vi "Selection ActionBuilder sections.vi"(6 "EC Query Array":T1[](array[typedef])=[enum."Is the EC Backing Pump ON?", enum."Does the EC Backing Pump have a fault?"], 7 "LB Query Array":T1[](array[typedef])=[enum."Is the LB Backing Pump ON?", enum."Does the LB Backing Pump have a fault?"], 9 "EC Command Array":T2[](array[typedef]), 10 "Chamber Selection":T3, 11 "LB Command Array":T2[](array[typedef])) -> (0 "Query Array out":T1[](array[typedef]), 3 "Command Array out":T2[](array[typedef]))   [LabVIEW 2011]
uses:
  Chamber Selection_typdef.ctl
  command_typdef.ctl
  action_typdef.ctl
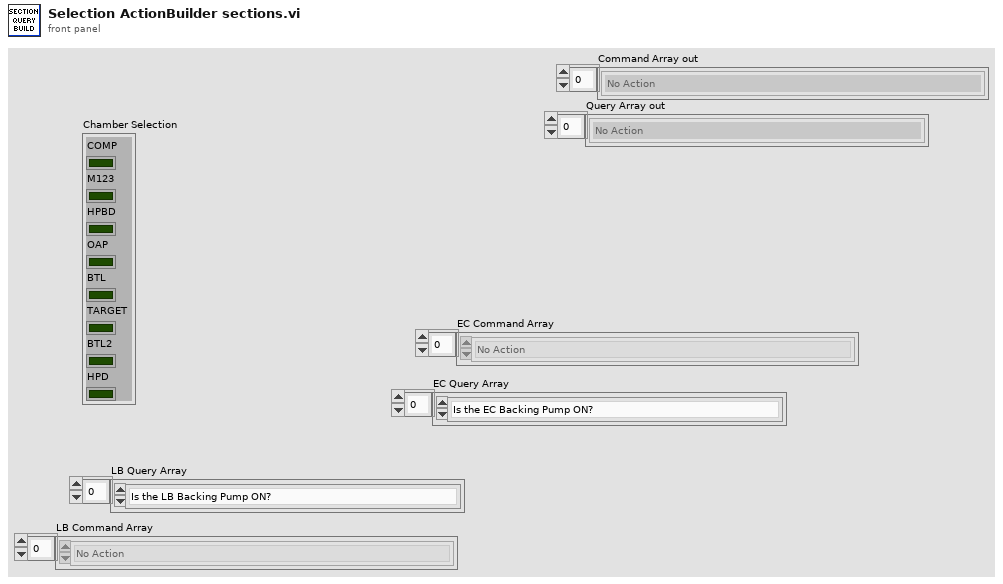
[diagram p1: front panel]
types:
  T1 = typedef "action_typdef.ctl" = enum16{"No Action", "Is EC GPM Mode ON?", "Is EC GPM Mode Off?", "Is EC GVM Mode ON?", "Is EC GVM Off?", "Is  EC GPM or GVM Mode ON?", "Is LB GPM Mode ON?", "Is LB GPM Mode Off?", "Is LB GVM Mode ON?", "Is LB GVM Mode Off?", "Is  LB GPM or GVM Mode ON?", "Is M123 Turbo Gate Valve Opened? ", "Is M123 Turbo Gate Valve Closed?", "Is OAP Turbo Gate Valve Opened?", "Is OAP Turbo Gate Valve Closed?", "Is BTLTurbo Gate Valve Opened?", "Is BTL Turbo Gate Valve Closed?", "Is TARGET Turbo Gate Valve 1Opened?", "Is TARGET1 Turbo Gate Valve Closed?", "Is TARGET Turbo Gate Valve 2 Opened?", "Is TAREGT2 Turbo Gate Valve Closed?", "Is BTL2 Turbo Gate Valve Opened?", "Is BTL2 Turbo Gate Valve Closed?", "Is HPD Turbo Gate Valve Opened?", "Is HPD Turbo Gate Valve Closed?", "Is COMP to M123 gate Valve Opened?", "Is COMP to M123 Valve Closed?", "Is HPBD Gate Valve Opened?", "Is HPBD Gate Valve Closed?", "Is M123 to OAP gate valve opened?", "Is M123 to OAP gate valve closed?", "Is OAP to BLT gate valve opened?", "Is OAP to BTL Gate Valve Closed?", "Is BLT to TARGET gate valve opened?", "Is BTL to TARGET Gate Valve Closed?", "Is TARGET to BLT2 gate valve opened?", "Is TARGET to BTL2 Gate Valve Closed?", "Is BLT2 to HPD gate valve opened?", "Is BTL2 to HPD Gate Valve Closed?", "Is COMP at Atmospheric Pressure?", "Is M123 at Atmospheric Pressure?", "Is BeamDump at Atmospheric Pressure?", "Is OAP at Atmospheric Pressure?", "Is BLT at Atmospheric Pressure", "Is TARGET at Atmospheric Pressure?", "Is BLT2 at Atmospheric Pressure?", "Is HPD at Atmospheric Pressure?", "Is the EC Roughing Pump ON?", "Is the EC Roughing Pump OFF?", "Does the EC Roughing Pump have a fault?", "Is the LB Roughing Pump ON?", "Is the LB Roughing Pump Off?", "Does the LB Roughing Pump have a fault?", "Is the EC Backing Pump ON?", "Is the EC Backing Pump OFF?", "Is the LB Backing Pump ON?", "Is the LB Backing Pump OFF?", "Does the EC Backing Pump have a fault?", "Does the LB Backing Pump have a fault?", "Is the EC Backing Pipe at Atmospheric Pressure", "Is the LB Backing Pipe at Atmospheric Pressure", "Is the EC Backing Manifold at Atmospheric Pressure", "s the LB Backing Manifold at Atmospheric Pressure?", "Is the EC Roughing Pipe at Atmospheric Pressure", "Is the LB Roughing Pipe at Atmospheric Pressure?", "Is the EC Roughing Manifold at Atmospheric Pressure", "Is the LB Roughing Manifold at Atmospheric Pressure", "Is LB Backing Manifold Valve Opened?", "Is EC Backing Manifold Valve Opened?", "Is LB Roughing Manifold Valve Opened?", "Is EC Roughing Manifold Valve Opened?", "Is COMP Roughing Valve Opened?", "Is M123 Roughing Valve Opened?", "Is M123 Roughing Valve Closed?", "Is OAP Roughing Valve Opened?", "Is OAP Roughing Valve Closed?", "Is HPBD Roughing Valve Opened?", "Is HPBD Roughing Valve Closed?", "Is BTL Roughing Valve Opened?", "Is BTL Roughing Valve Closed?", "Is TARGET Roughing Valve Opened?", "Is TARGET Roughing Valve Closed?", "Is BTL2 Roughing Valve Opened?", "Is BTL2 Roughing Valve Closed?", "Is HPD Roughing Valve Opened?", "Is HPD Roughing Valve Closed?", "Is COMP Turbo Backing Valve Opened?", "Is M123 Turbo Backing Valve Opened", "Is HPBD Turbo Backing Valve Opened?", "Is OAP Turbo Backing Valve Opened?", "Is BTL Turbo Backing Valve Opened?", "Is TARGET1 Turbo Backing Valve Opened?", "Is TARGET2 Turbo Backing Valve Opened?", "Is BTL2 Turbo Backing Valve Opened?", "Is HPD Turbo Backing Valve Opened?", "Is M123 Backing at MID-VAC?", "Is OAP Backing at MID-VAC?", "Is TARGET1 Backing at MID-VAC?", "Is TARGET2 Backing at MID-VAC?", "Is BTL Backing at MID-VAC?", "Is BTL2 Backing at MID-VAC?", "Is HPD Backing at MID-VAC?", "Is M123 Turbo in Normal Operation", "Is COMP Turbo in Normal Operation", "Is OAP Turbo in Normal Operation", "Is BTL Turbo in Normal Operation", "Is TARGET1 Turbo in Normal Operation", "Is TARGET2 Turbo in Normal Operation", "Is BTL2 Turbo in Normal Operation", "Is HPD Turbo in Normal Operation", "Is M123 at MID-VAC?", "Is OAP at MID-VAC?", "Is COMP at MID-VAC?", "Is BTL at MID-VAC?", "Is TARGET at MID-VAC?", "Is BTL2 at MID-VAC?", "Is HPD at MID-VAC?"}
  T2 = typedef "command_typdef.ctl" = enum16{"No Action", "Set GPM Mode LB", "EXIT GPM Mode LB", "Set GPM Mode EC", "EXIT GPM Mode EC", "Set GVM mode LB", "Set GVM Mode EC", "Open LB Backing Valve", "Open EC Backing Valve", "Open EC Roughing Valve", "Open LB Roughing Valve", "Open M123 Roughing Valve", "Close M123 Roughing Valve", "Open Compressor Roughing Valve", "Close Compressor Roughing Valve", "Open BeamDump Roughing Valve", "Close BeamDump Roughing Valve", "Open OAP Roughing Valve", "Close OAP Roughing Valve", "Open BTL Roughing Valve", "Close BTL Roughing Valve", "Open Target Roughing Valve", "Close Target Roughing Valve", "Open BTL2 Roughing Valve", "Close BTL2 Roughing Valve", "Open HPD Roughing Valve", "Close HPD Roughing Valve", "LB Start Roughing Pump ", "EC Start Roughing Pump", "Open COMP Turbo Backing Valve", "Open M123 Turbo Backing Valve", "Open OAP Turbo Backing Valve", "Open HPBD Turbo Backing Valve", "Open BLT Turbo Backing Valve", "Open TARGET1 Turbo Backing Valve", "Open TARGET2 Turbo Backing Valve", "Open BLT2 Turbo Backing Valve", "Open HPD Turbo Backing Valve", "LB Start Turbo Backing Pump", "EC Start Turbo Backing Pump", "Start COMP Turbo Pump", "Start M123 Turbo Pump", "Start OAP Turbo Pump", "Start BTL Turbo Pump", "Start TARGET1 Turbo Pump", "Start TARGET2 Turbo Pump", "Start BTL2 Turbo Pump", "Start HPD Turbo Pump", "Open COMP Turbo Gate Valve", "Open M123 Turbo Gate Valve", "Open OAP Turbo Gate Valve", "Open BTL Turbo Gate Valve", "Open TARGET1 Turbo Gate Valve", "Open TARGET2 Turbo Gate Valve", "Open BTL2 Turbo Gate Valve", "Open HPD Turbo Gate Valve"}
  T3 = typedef "Chamber Selection_typdef.ctl" = cluster{"COMP":bool, "M123":bool, "HPBD":bool, "OAP":bool, "BTL":bool, "TARGET":bool, "BTL2":bool, "HPD":bool}
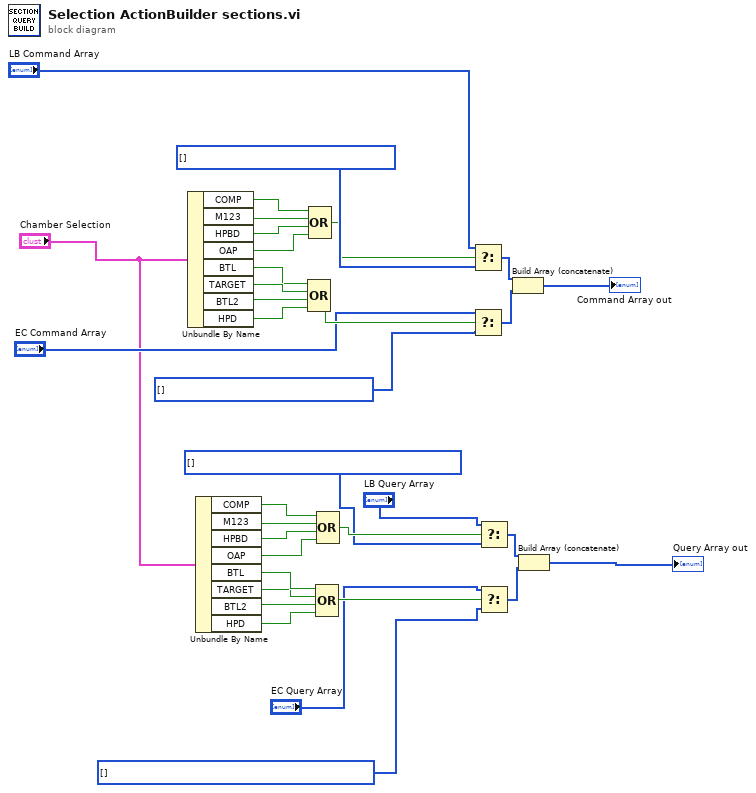
[diagram p0: block diagram]
diagram:
  w2 = T1[] [] items=["No Action", "Is EC GPM Mode ON?", "Is EC GPM Mode Off?", "Is EC GVM Mode ON?", "Is EC GVM Off?", "Is  EC GPM or GVM Mode ON?", "Is LB GPM Mode ON?", "Is LB GPM Mode Off?", "Is LB GVM Mode ON?", "Is LB GVM Mode Off?", "Is  LB GPM or GVM Mode ON?", "Is M123 Turbo Gate Valve Opened? ", "Is M123 Turbo Gate Valve Closed?", "Is OAP Turbo Gate Valve Opened?", "Is OAP Turbo Gate Valve Closed?", "Is BTLTurbo Gate Valve Opened?", "Is BTL Turbo Gate Valve Closed?", "Is TARGET Turbo Gate Valve 1Opened?", "Is TARGET1 Turbo Gate Valve Closed?", "Is TARGET Turbo Gate Valve 2 Opened?", "Is TAREGT2 Turbo Gate Valve Closed?", "Is BTL2 Turbo Gate Valve Opened?", "Is BTL2 Turbo Gate Valve Closed?", "Is HPD Turbo Gate Valve Opened?", "Is HPD Turbo Gate Valve Closed?", "Is COMP to M123 gate Valve Opened?", "Is COMP to M123 Valve Closed?", "Is HPBD Gate Valve Opened?", "Is HPBD Gate Valve Closed?", "Is M123 to OAP gate valve opened?", "Is M123 to OAP gate valve closed?", "Is OAP to BLT gate valve opened?", "Is OAP to BTL Gate Valve Closed?", "Is BLT to TARGET gate valve opened?", "Is BTL to TARGET Gate Valve Closed?", "Is TARGET to BLT2 gate valve opened?", "Is TARGET to BTL2 Gate Valve Closed?", "Is BLT2 to HPD gate valve opened?", "Is BTL2 to HPD Gate Valve Closed?", "Is COMP at Atmospheric Pressure?", "Is M123 at Atmospheric Pressure?", "Is BeamDump at Atmospheric Pressure?", "Is OAP at Atmospheric Pressure?", "Is BLT at Atmospheric Pressure", "Is TARGET at Atmospheric Pressure?", "Is BLT2 at Atmospheric Pressure?", "Is HPD at Atmospheric Pressure?", "Is the EC Roughing Pump ON?", "Is the EC Roughing Pump OFF?", "Does the EC Roughing Pump have a fault?", "Is the LB Roughing Pump ON?", "Is the LB Roughing Pump Off?", "Does the LB Roughing Pump have a fault?", "Is the EC Backing Pump ON?", "Is the EC Backing Pump OFF?", "Is the LB Backing Pump ON?", "Is the LB Backing Pump OFF?", "Does the EC Backing Pump have a fault?", "Does the LB Backing Pump have a fault?", "Is the EC Backing Pipe at Atmospheric Pressure", "Is the LB Backing Pipe at Atmospheric Pressure", "Is the EC Backing Manifold at Atmospheric Pressure", "s the LB Backing Manifold at Atmospheric Pressure?", "Is the EC Roughing Pipe at Atmospheric Pressure", "Is the LB Roughing Pipe at Atmospheric Pressure?", "Is the EC Roughing Manifold at Atmospheric Pressure", "Is the LB Roughing Manifold at Atmospheric Pressure", "Is LB Backing Manifold Valve Opened?", "Is EC Backing Manifold Valve Opened?", "Is LB Roughing Manifold Valve Opened?", "Is EC Roughing Manifold Valve Opened?", "Is COMP Roughing Valve Opened?", "Is M123 Roughing Valve Opened?", "Is M123 Roughing Valve Closed?", "Is OAP Roughing Valve Opened?", "Is OAP Roughing Valve Closed?", "Is HPBD Roughing Valve Opened?", "Is HPBD Roughing Valve Closed?", "Is BTL Roughing Valve Opened?", "Is BTL Roughing Valve Closed?", "Is TARGET Roughing Valve Opened?", "Is TARGET Roughing Valve Closed?", "Is BTL2 Roughing Valve Opened?", "Is BTL2 Roughing Valve Closed?", "Is HPD Roughing Valve Opened?", "Is HPD Roughing Valve Closed?", "Is COMP Turbo Backing Valve Opened?", "Is M123 Turbo Backing Valve Opened", "Is HPBD Turbo Backing Valve Opened?", "Is OAP Turbo Backing Valve Opened?", "Is BTL Turbo Backing Valve Opened?", "Is TARGET1 Turbo Backing Valve Opened?", "Is TARGET2 Turbo Backing Valve Opened?", "Is BTL2 Turbo Backing Valve Opened?", "Is HPD Turbo Backing Valve Opened?", "Is M123 Backing at MID-VAC?", "Is OAP Backing at MID-VAC?", "Is TARGET1 Backing at MID-VAC?", "Is TARGET2 Backing at MID-VAC?", "Is BTL Backing at MID-VAC?", "Is BTL2 Backing at MID-VAC?", "Is HPD Backing at MID-VAC?", "Is M123 Turbo in Normal Operation", "Is COMP Turbo in Normal Operation", "Is OAP Turbo in Normal Operation", "Is BTL Turbo in Normal Operation", "Is TARGET1 Turbo in Normal Operation", "Is TARGET2 Turbo in Normal Operation", "Is BTL2 Turbo in Normal Operation", "Is HPD Turbo in Normal Operation", "Is M123 at MID-VAC?", "Is OAP at MID-VAC?", "Is COMP at MID-VAC?", "Is BTL at MID-VAC?", "Is TARGET at MID-VAC?", "Is BTL2 at MID-VAC?", "Is HPD at MID-VAC?"]
  w3 = T1[] [] items=["No Action", "Is EC GPM Mode ON?", "Is EC GPM Mode Off?", "Is EC GVM Mode ON?", "Is EC GVM Off?", "Is  EC GPM or GVM Mode ON?", "Is LB GPM Mode ON?", "Is LB GPM Mode Off?", "Is LB GVM Mode ON?", "Is LB GVM Mode Off?", "Is  LB GPM or GVM Mode ON?", "Is M123 Turbo Gate Valve Opened? ", "Is M123 Turbo Gate Valve Closed?", "Is OAP Turbo Gate Valve Opened?", "Is OAP Turbo Gate Valve Closed?", "Is BTLTurbo Gate Valve Opened?", "Is BTL Turbo Gate Valve Closed?", "Is TARGET Turbo Gate Valve 1Opened?", "Is TARGET1 Turbo Gate Valve Closed?", "Is TARGET Turbo Gate Valve 2 Opened?", "Is TAREGT2 Turbo Gate Valve Closed?", "Is BTL2 Turbo Gate Valve Opened?", "Is BTL2 Turbo Gate Valve Closed?", "Is HPD Turbo Gate Valve Opened?", "Is HPD Turbo Gate Valve Closed?", "Is COMP to M123 gate Valve Opened?", "Is COMP to M123 Valve Closed?", "Is HPBD Gate Valve Opened?", "Is HPBD Gate Valve Closed?", "Is M123 to OAP gate valve opened?", "Is M123 to OAP gate valve closed?", "Is OAP to BLT gate valve opened?", "Is OAP to BTL Gate Valve Closed?", "Is BLT to TARGET gate valve opened?", "Is BTL to TARGET Gate Valve Closed?", "Is TARGET to BLT2 gate valve opened?", "Is TARGET to BTL2 Gate Valve Closed?", "Is BLT2 to HPD gate valve opened?", "Is BTL2 to HPD Gate Valve Closed?", "Is COMP at Atmospheric Pressure?", "Is M123 at Atmospheric Pressure?", "Is BeamDump at Atmospheric Pressure?", "Is OAP at Atmospheric Pressure?", "Is BLT at Atmospheric Pressure", "Is TARGET at Atmospheric Pressure?", "Is BLT2 at Atmospheric Pressure?", "Is HPD at Atmospheric Pressure?", "Is the EC Roughing Pump ON?", "Is the EC Roughing Pump OFF?", "Does the EC Roughing Pump have a fault?", "Is the LB Roughing Pump ON?", "Is the LB Roughing Pump Off?", "Does the LB Roughing Pump have a fault?", "Is the EC Backing Pump ON?", "Is the EC Backing Pump OFF?", "Is the LB Backing Pump ON?", "Is the LB Backing Pump OFF?", "Does the EC Backing Pump have a fault?", "Does the LB Backing Pump have a fault?", "Is the EC Backing Pipe at Atmospheric Pressure", "Is the LB Backing Pipe at Atmospheric Pressure", "Is the EC Backing Manifold at Atmospheric Pressure", "s the LB Backing Manifold at Atmospheric Pressure?", "Is the EC Roughing Pipe at Atmospheric Pressure", "Is the LB Roughing Pipe at Atmospheric Pressure?", "Is the EC Roughing Manifold at Atmospheric Pressure", "Is the LB Roughing Manifold at Atmospheric Pressure", "Is LB Backing Manifold Valve Opened?", "Is EC Backing Manifold Valve Opened?", "Is LB Roughing Manifold Valve Opened?", "Is EC Roughing Manifold Valve Opened?", "Is COMP Roughing Valve Opened?", "Is M123 Roughing Valve Opened?", "Is M123 Roughing Valve Closed?", "Is OAP Roughing Valve Opened?", "Is OAP Roughing Valve Closed?", "Is HPBD Roughing Valve Opened?", "Is HPBD Roughing Valve Closed?", "Is BTL Roughing Valve Opened?", "Is BTL Roughing Valve Closed?", "Is TARGET Roughing Valve Opened?", "Is TARGET Roughing Valve Closed?", "Is BTL2 Roughing Valve Opened?", "Is BTL2 Roughing Valve Closed?", "Is HPD Roughing Valve Opened?", "Is HPD Roughing Valve Closed?", "Is COMP Turbo Backing Valve Opened?", "Is M123 Turbo Backing Valve Opened", "Is HPBD Turbo Backing Valve Opened?", "Is OAP Turbo Backing Valve Opened?", "Is BTL Turbo Backing Valve Opened?", "Is TARGET1 Turbo Backing Valve Opened?", "Is TARGET2 Turbo Backing Valve Opened?", "Is BTL2 Turbo Backing Valve Opened?", "Is HPD Turbo Backing Valve Opened?", "Is M123 Backing at MID-VAC?", "Is OAP Backing at MID-VAC?", "Is TARGET1 Backing at MID-VAC?", "Is TARGET2 Backing at MID-VAC?", "Is BTL Backing at MID-VAC?", "Is BTL2 Backing at MID-VAC?", "Is HPD Backing at MID-VAC?", "Is M123 Turbo in Normal Operation", "Is COMP Turbo in Normal Operation", "Is OAP Turbo in Normal Operation", "Is BTL Turbo in Normal Operation", "Is TARGET1 Turbo in Normal Operation", "Is TARGET2 Turbo in Normal Operation", "Is BTL2 Turbo in Normal Operation", "Is HPD Turbo in Normal Operation", "Is M123 at MID-VAC?", "Is OAP at MID-VAC?", "Is COMP at MID-VAC?", "Is BTL at MID-VAC?", "Is TARGET at MID-VAC?", "Is BTL2 at MID-VAC?", "Is HPD at MID-VAC?"]
  w31 = T2[] [] items=["No Action", "Set GPM Mode LB", "EXIT GPM Mode LB", "Set GPM Mode EC", "EXIT GPM Mode EC", "Set GVM mode LB", "Set GVM Mode EC", "Open LB Backing Valve", "Open EC Backing Valve", "Open EC Roughing Valve", "Open LB Roughing Valve", "Open M123 Roughing Valve", "Close M123 Roughing Valve", "Open Compressor Roughing Valve", "Close Compressor Roughing Valve", "Open BeamDump Roughing Valve", "Close BeamDump Roughing Valve", "Open OAP Roughing Valve", "Close OAP Roughing Valve", "Open BTL Roughing Valve", "Close BTL Roughing Valve", "Open Target Roughing Valve", "Close Target Roughing Valve", "Open BTL2 Roughing Valve", "Close BTL2 Roughing Valve", "Open HPD Roughing Valve", "Close HPD Roughing Valve", "LB Start Roughing Pump ", "EC Start Roughing Pump", "Open COMP Turbo Backing Valve", "Open M123 Turbo Backing Valve", "Open OAP Turbo Backing Valve", "Open HPBD Turbo Backing Valve", "Open BLT Turbo Backing Valve", "Open TARGET1 Turbo Backing Valve", "Open TARGET2 Turbo Backing Valve", "Open BLT2 Turbo Backing Valve", "Open HPD Turbo Backing Valve", "LB Start Turbo Backing Pump", "EC Start Turbo Backing Pump", "Start COMP Turbo Pump", "Start M123 Turbo Pump", "Start OAP Turbo Pump", "Start BTL Turbo Pump", "Start TARGET1 Turbo Pump", "Start TARGET2 Turbo Pump", "Start BTL2 Turbo Pump", "Start HPD Turbo Pump", "Open COMP Turbo Gate Valve", "Open M123 Turbo Gate Valve", "Open OAP Turbo Gate Valve", "Open BTL Turbo Gate Valve", "Open TARGET1 Turbo Gate Valve", "Open TARGET2 Turbo Gate Valve", "Open BTL2 Turbo Gate Valve", "Open HPD Turbo Gate Valve"]
  w29 = T2[] [] items=["No Action", "Set GPM Mode LB", "EXIT GPM Mode LB", "Set GPM Mode EC", "EXIT GPM Mode EC", "Set GVM mode LB", "Set GVM Mode EC", "Open LB Backing Valve", "Open EC Backing Valve", "Open EC Roughing Valve", "Open LB Roughing Valve", "Open M123 Roughing Valve", "Close M123 Roughing Valve", "Open Compressor Roughing Valve", "Close Compressor Roughing Valve", "Open BeamDump Roughing Valve", "Close BeamDump Roughing Valve", "Open OAP Roughing Valve", "Close OAP Roughing Valve", "Open BTL Roughing Valve", "Close BTL Roughing Valve", "Open Target Roughing Valve", "Close Target Roughing Valve", "Open BTL2 Roughing Valve", "Close BTL2 Roughing Valve", "Open HPD Roughing Valve", "Close HPD Roughing Valve", "LB Start Roughing Pump ", "EC Start Roughing Pump", "Open COMP Turbo Backing Valve", "Open M123 Turbo Backing Valve", "Open OAP Turbo Backing Valve", "Open HPBD Turbo Backing Valve", "Open BLT Turbo Backing Valve", "Open TARGET1 Turbo Backing Valve", "Open TARGET2 Turbo Backing Valve", "Open BLT2 Turbo Backing Valve", "Open HPD Turbo Backing Valve", "LB Start Turbo Backing Pump", "EC Start Turbo Backing Pump", "Start COMP Turbo Pump", "Start M123 Turbo Pump", "Start OAP Turbo Pump", "Start BTL Turbo Pump", "Start TARGET1 Turbo Pump", "Start TARGET2 Turbo Pump", "Start BTL2 Turbo Pump", "Start HPD Turbo Pump", "Open COMP Turbo Gate Valve", "Open M123 Turbo Gate Valve", "Open OAP Turbo Gate Valve", "Open BTL Turbo Gate Valve", "Open TARGET1 Turbo Gate Valve", "Open TARGET2 Turbo Gate Valve", "Open BTL2 Turbo Gate Valve", "Open HPD Turbo Gate Valve"]
  n1 = Unbundle By Name("Chamber Selection") -> ("COMP"=w19:bool, "M123"=w20:bool, "HPBD"=w21:bool, "OAP"=w22:bool, "BTL"=w23:bool, "TARGET"=w24:bool, "BTL2"=w25:bool, "HPD"=w26:bool)
  n2 = Unbundle By Name("Chamber Selection") -> ("COMP"=w18:bool, "M123"=w17:bool, "HPBD"=w16:bool, "OAP"=w15:bool, "BTL"=w14:bool, "TARGET"=w13:bool, "BTL2"=w12:bool, "HPD"=w11:bool)
  n3 = Compound Arithmetic op=OR(w23, w24, w25, w26) -> (w32:bool)
  n4 = Compound Arithmetic op=OR(w19, w20, w21, w22) -> (w27:bool)
  n5 = Compound Arithmetic op=OR(w14, w13, w12, w11) -> (w9:bool)
  n6 = Compound Arithmetic op=OR(w18, w17, w16, w15) -> (w10:bool)
  n7 = Select(t="LB Command Array", s=w27, f=w29) -> (s? t:f=w33:T2[])
  n8 = Select(t="EC Command Array", s=w32, f=w31) -> (s? t:f=w34:T2[])
  n9 = Select(t="LB Query Array", s=w10, f=w3) -> (s? t:f=w8:T1[])
  n10 = Select(t="EC Query Array", s=w9, f=w2) -> (s? t:f=w7:T1[])
  n11 = Build Array (concatenate)(w33, w34) -> (→"Command Array out":T2[])
  n12 = Build Array (concatenate)(w8, w7) -> (→"Query Array out":T1[])
